vi "Update Controls.vi"(8 "error in":errorcluster, 10 "MHL References":T2, 11 "MHL Status":T1) -> (0 "error out":errorcluster)   [LabVIEW 2014]
uses:
  controls/MHL References.ctl
  controls/MHL Status.ctl
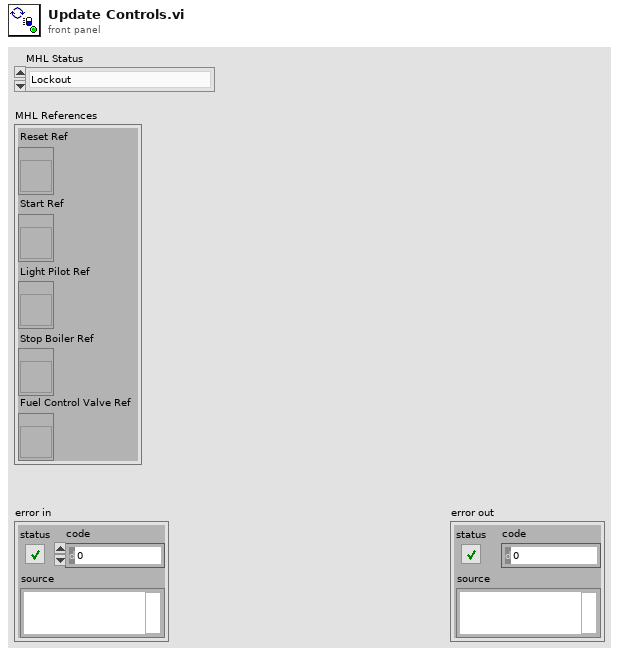
[diagram p1: front panel]
types:
  T1 = typedef "MHL Status.ctl" = enum16{"Lockout", "Ready", "Pre-Purge", "Pre-Purge Complete", "Pilot On", "Boiler Running", "Shutdown", "Purge"}
  T2 = typedef "MHL References.ctl" = cluster{"Reset Ref":refnum<vi>, "Start Ref":refnum<vi>, "Light Pilot Ref":refnum<vi>, "Stop Boiler Ref":refnum<vi>, "Fuel Control Valve Ref":refnum<vi>}
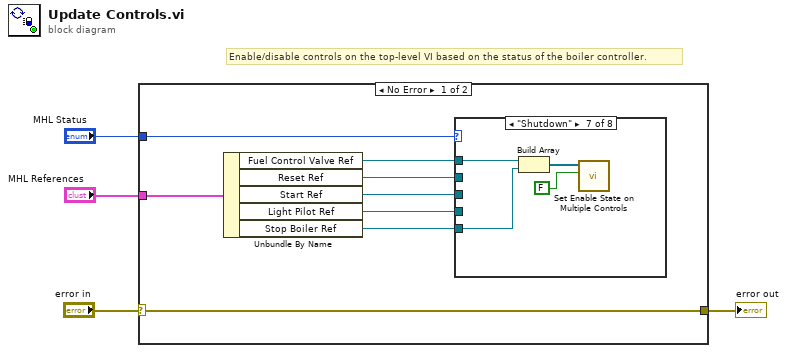
[diagram p0: block diagram]
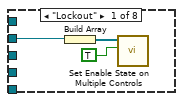
[diagram p2: hidden frame]
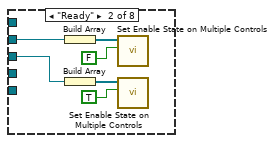
[diagram p3: hidden frame]
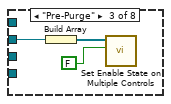
[diagram p4: hidden frame]
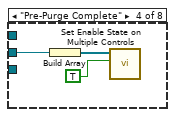
[diagram p5: hidden frame]
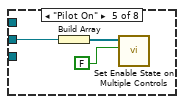
[diagram p6: hidden frame]
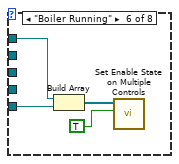
[diagram p7: hidden frame]
diagram:
  # "Enable/disable controls on the top-level VI based on the status of the boiler controller."
  n1 = case shown="No Error" "error in" {
    selector: "error in" -> [w5 w39]
    tunnel: "MHL References" -> [w12 _]
    tunnel: "MHL Status" -> [w11 _]
    tunnel: [w5 w39] -> w1
    frame No Error {
      n2 = Unbundle By Name(w12) -> ("Fuel Control Valve Ref"=w10:refnum<vi>, "Reset Ref"=w9:refnum<vi>, "Start Ref"=w8:refnum<vi>, "Light Pilot Ref"=w7:refnum<vi>, "Stop Boiler Ref"=w6:refnum<vi>)
      n3 = case shown="\"Shutdown\"" w11 {
        tunnel: w6 -> [_ _ _ _ _ w32 w36 _]
        tunnel: w7 -> [_ _ _ w25 w28 _ _ _]
        tunnel: w8 -> [_ w18 w24 _ _ _ _ _]
        tunnel: w9 -> [w13 w21 _ _ _ _ _ _]
        tunnel: w10 -> [_ _ _ _ _ w31 w35 _]
        frame "Lockout" {
          n4 = Build Array(w13) -> (w15:refnum<vi>[])
          n5 = call "Set Enable State on Multiple Controls.vi"("Enable?"=TRUE, "Controls"=w15) -> ()  [unwired: 10 in]
        }
        frame "Ready" {
          n6 = Build Array(w21) -> (w20:refnum<vi>[])
          n7 = Build Array(w18) -> (w17:refnum<vi>[])
          n8 = call "Set Enable State on Multiple Controls.vi"("Enable?"=FALSE, "Controls"=w20) -> ()  [unwired: 10 in]
          n9 = call "Set Enable State on Multiple Controls.vi"("Enable?"=TRUE, "Controls"=w17) -> ()  [unwired: 10 in]
        }
        frame "Pre-Purge" {
          n10 = Build Array(w24) -> (w23:refnum<vi>[])
          n11 = call "Set Enable State on Multiple Controls.vi"("Enable?"=FALSE, "Controls"=w23) -> ()  [unwired: 10 in]
        }
        frame "Pre-Purge Complete" {
          n12 = Build Array(w25) -> (w27:refnum<vi>[])
          n13 = call "Set Enable State on Multiple Controls.vi"("Enable?"=TRUE, "Controls"=w27) -> ()  [unwired: 10 in]
        }
        frame "Pilot On" {
          n14 = Build Array(w28) -> (w30:refnum<vi>[])
          n15 = call "Set Enable State on Multiple Controls.vi"("Enable?"=FALSE, "Controls"=w30) -> ()  [unwired: 10 in]
        }
        frame "Boiler Running" {
          n16 = Build Array(w31, w32) -> (w34:refnum<vi>[])
          n17 = call "Set Enable State on Multiple Controls.vi"("Enable?"=TRUE, "Controls"=w34) -> ()  [unwired: 10 in]
        }
        frame "Shutdown" {
          n18 = Build Array(w35, w36) -> (w38:refnum<vi>[])
          n19 = call "Set Enable State on Multiple Controls.vi"("Enable?"=FALSE, "Controls"=w38) -> ()  [unwired: 10 in]
        }
        frame "Purge" {
          # "No Action"
        }
      }
    }
    frame Error {
    }
  }
  "error out" <- w1
